vi "Select Popup_General_UI.vi"(8 "error in (no error)":errorcluster, 9 "Self Enqueuer":refnum<class "Message Enqueuer.lvclass">, 11 "ZenGage v3.0 UI in":refnum<class "ZenGage v3.0 UI.lvclass">) -> (0 "error out":errorcluster, 1 "Selection Cancelled?":bool, 2 "JSON Read?":bool, 3 "ZenGage v3.0 UI out":refnum<class "ZenGage v3.0 UI.lvclass">, 5 "Max limits":cluster{"Production max":i32, "Reel max":i32})   [LabVIEW 2015, in "ZenGage v3.0 UI.lvclass"]
uses:
  ZenGage v3.0 UI.lvclass
  <vilib>/ActorFramework/Message Enqueuer/Message Enqueuer.lvclass
  ZenGage v3.0 UI.lvclass/ZenGage v3.0 UI.ctl
  Inspection Statemachine/Inspection Statemachine Messages/Load Selected Part_SM Msg/Load Selected Part_SM Msg.lvclass/Load Selected Part_SM Msg.ctl
  <vilib>/ActorFramework/Message Enqueuer/Message Enqueuer.lvclass/Message Enqueuer.ctl
  <vilib>/ActorFramework/Message Enqueuer/Enqueue.vi
  <vilib>/ActorFramework/Message Priority Queue/Priority Enqueue.vi
  Inspection Statemachine/Inspection Statemachine Messages/Load Selected Part_SM Msg/Load Selected Part_SM Msg.lvclass
panel:
  in  "cancel button":bool
  out "Dialog Box out":string="             SELECT A PART TO INSPECT"
  in  "Combo Box":string(combo)
  in  "String":string
  in  "Numeric Control":dbl
  in  "OK Button":bool
  in  "OK Button":bool
  in  "ORDER NUMBER":dbl
  in  "ORDER NUMBER":dbl
  in  "OPERATOR ID":string
  in  "ORDER NUMBER":dbl
  in  "PART NAME":string(combo)
  # "Select a part to Inspect"
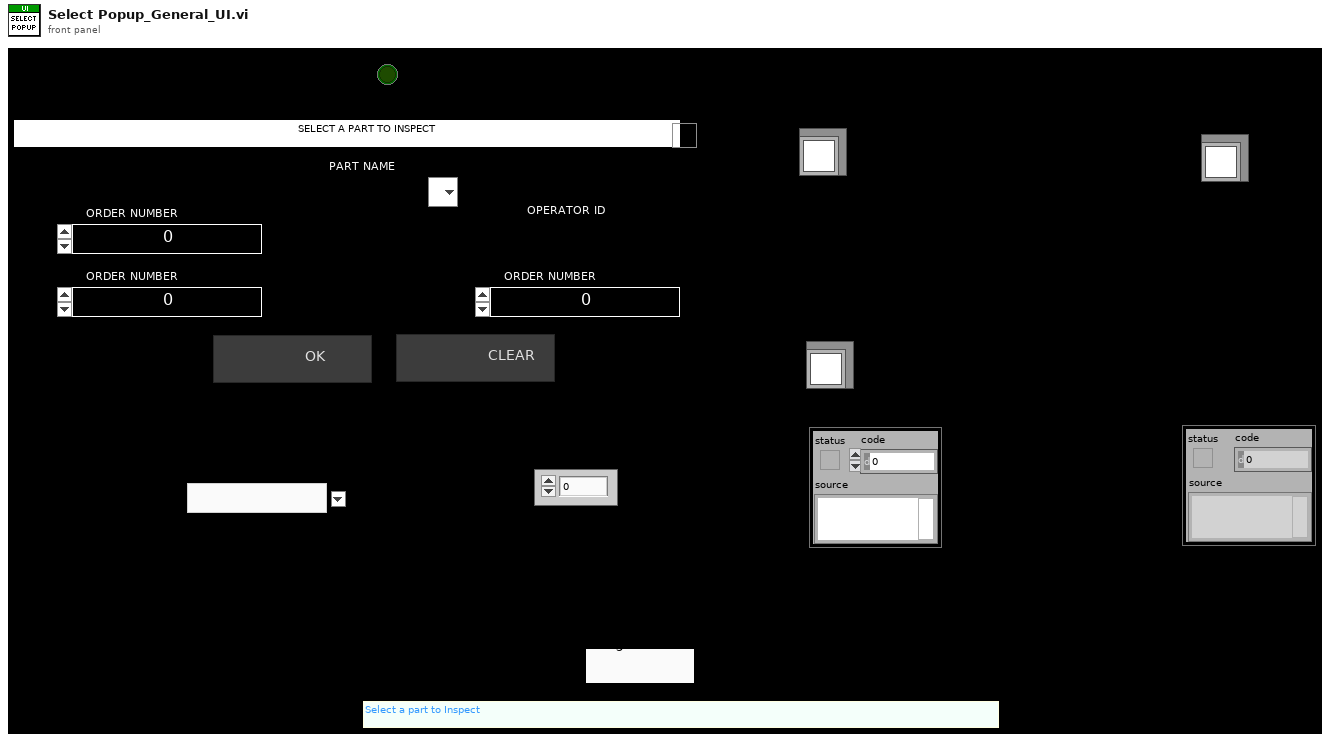
[diagram p1: front panel]
types:
  T1 = enum32{"Invalid", "Standard", "Closed", "Hidden", "Minimized", "Maximized"}
  T2 = cluster{"Part Name":string, "Total Counts":u64, "Connectors in Reel":u64, "Stamping machine ID":u8, "Operator Code":string, "Rack-1 ":bool, "Rack-2 ":bool, "Number of Racks":i32}
  T3 = cluster{"Part Name":string, "Operator Number":string, "Order Number":string}
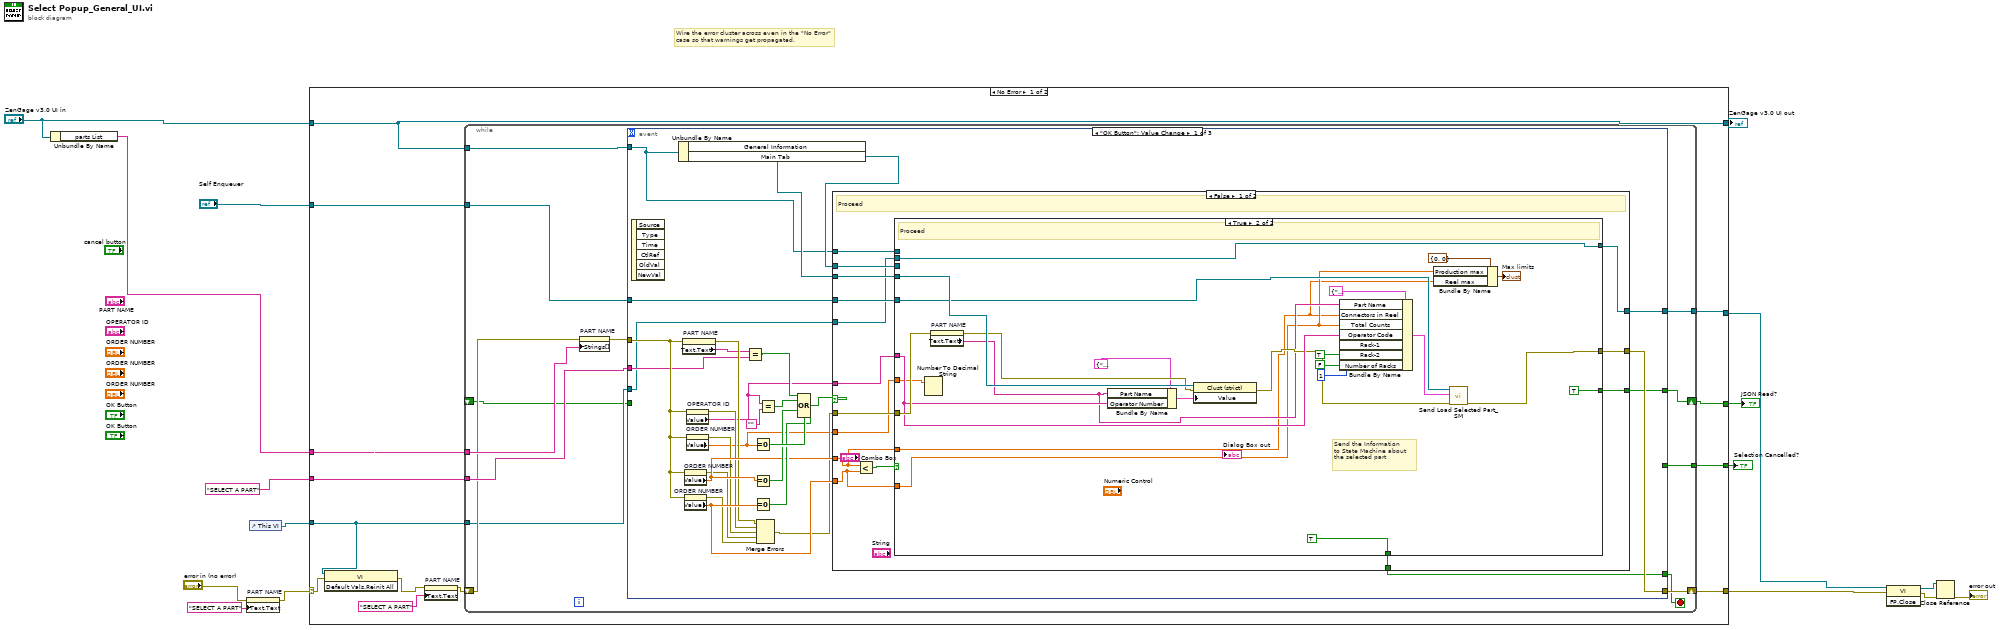
[diagram p0: block diagram]
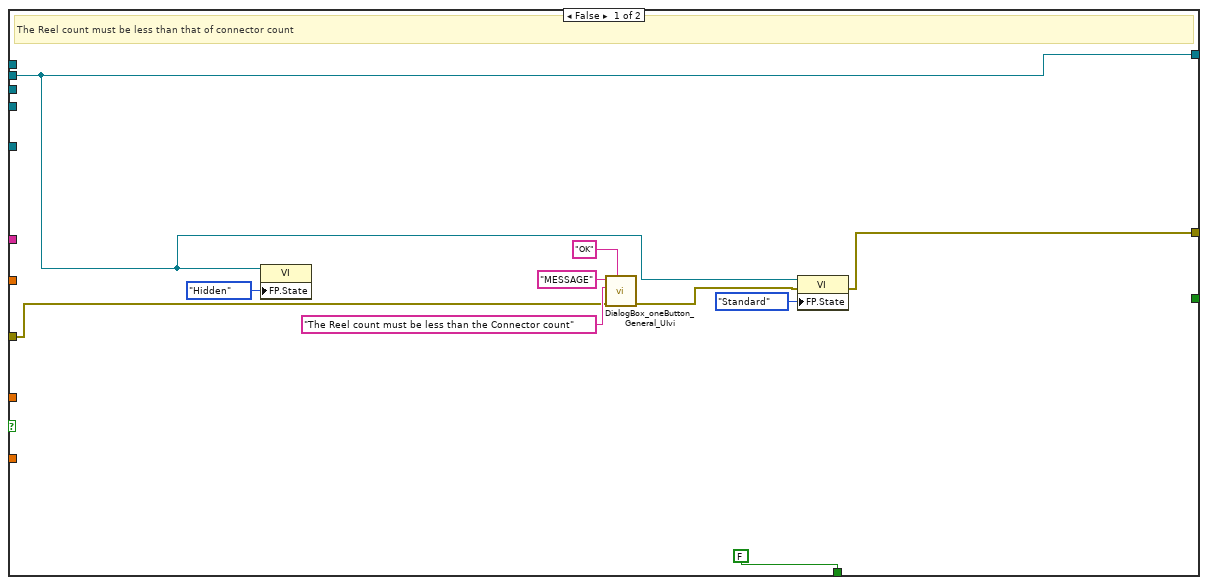
[diagram p2: hidden frame]
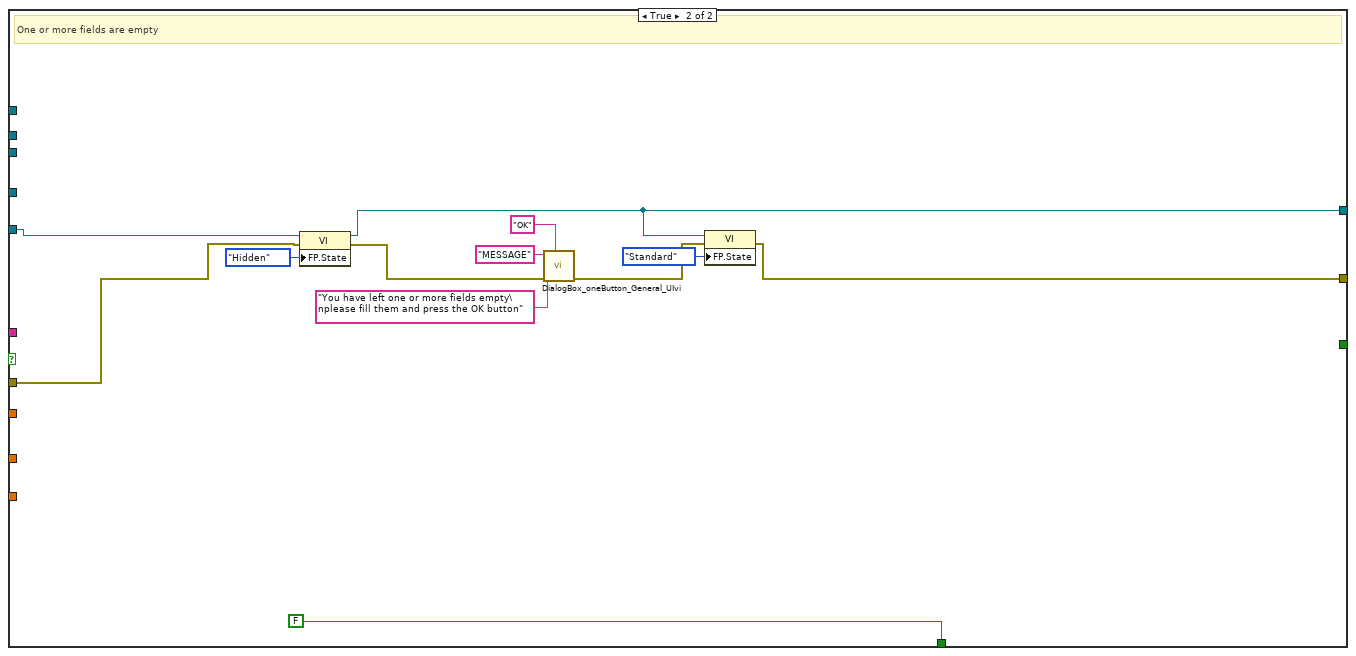
[diagram p3: hidden frame]
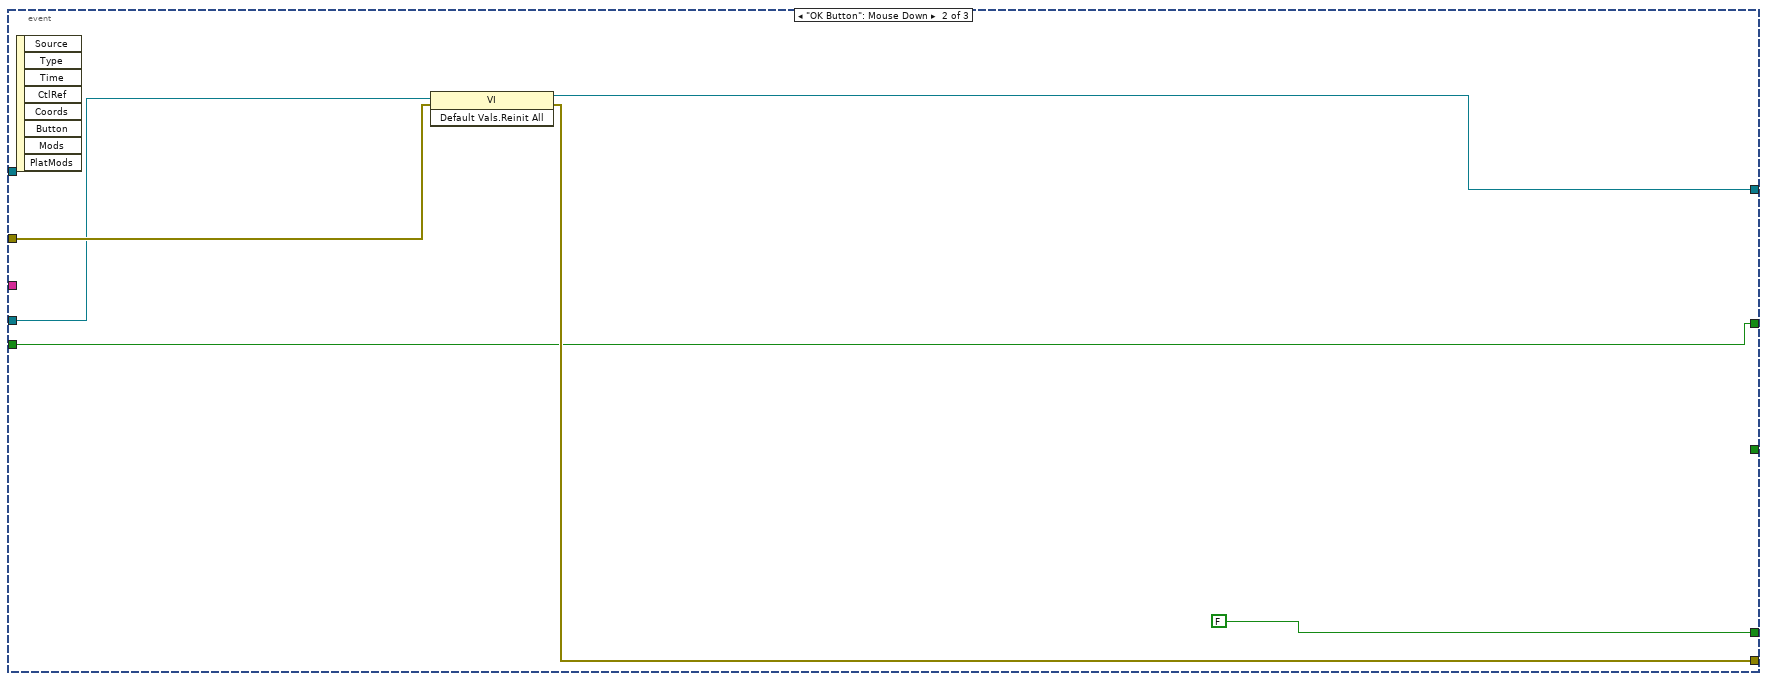
[diagram p4: hidden frame]
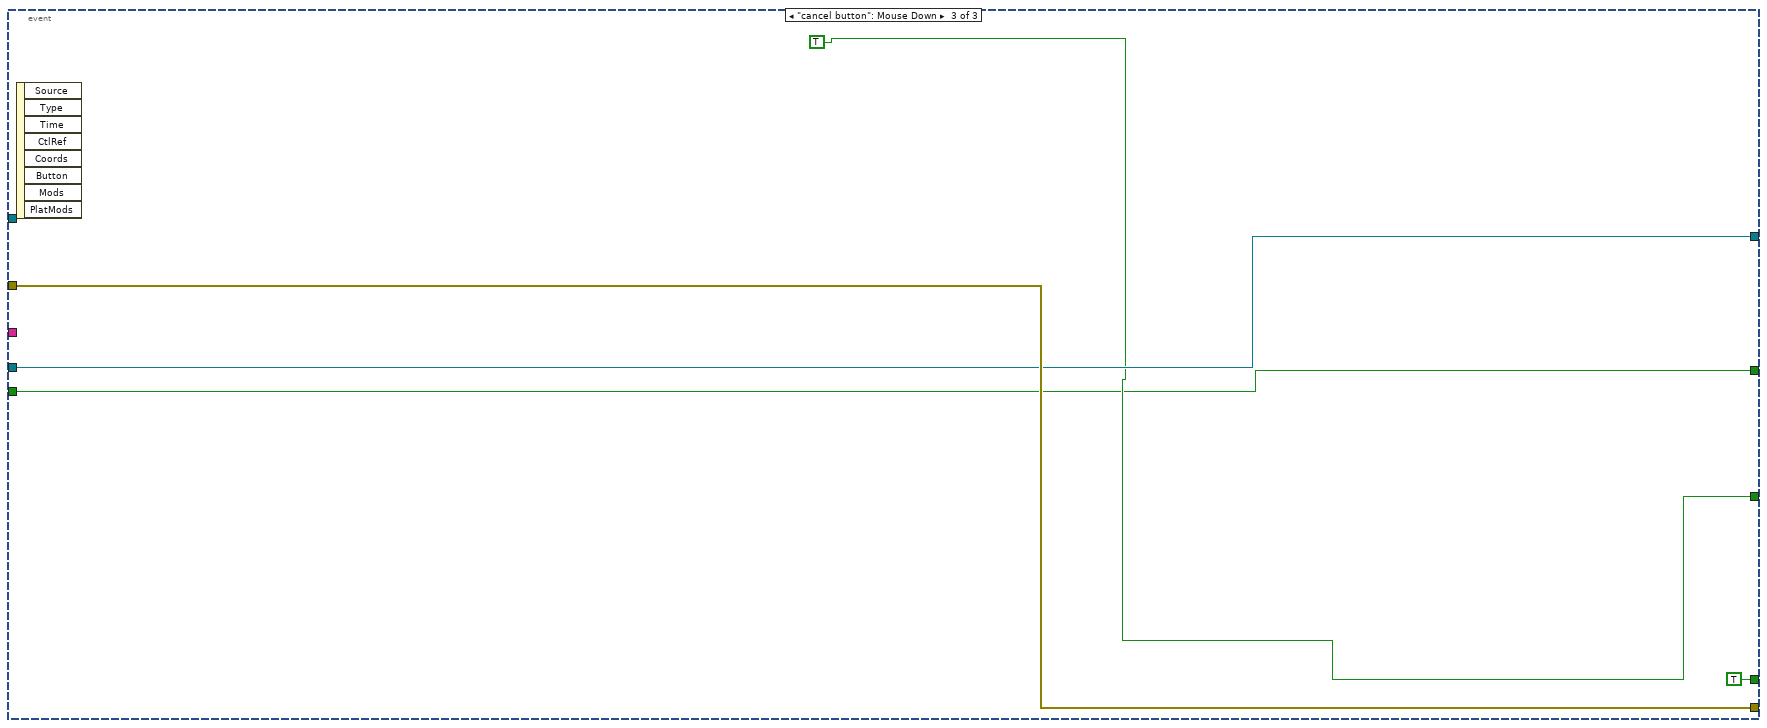
[diagram p5: hidden frame]
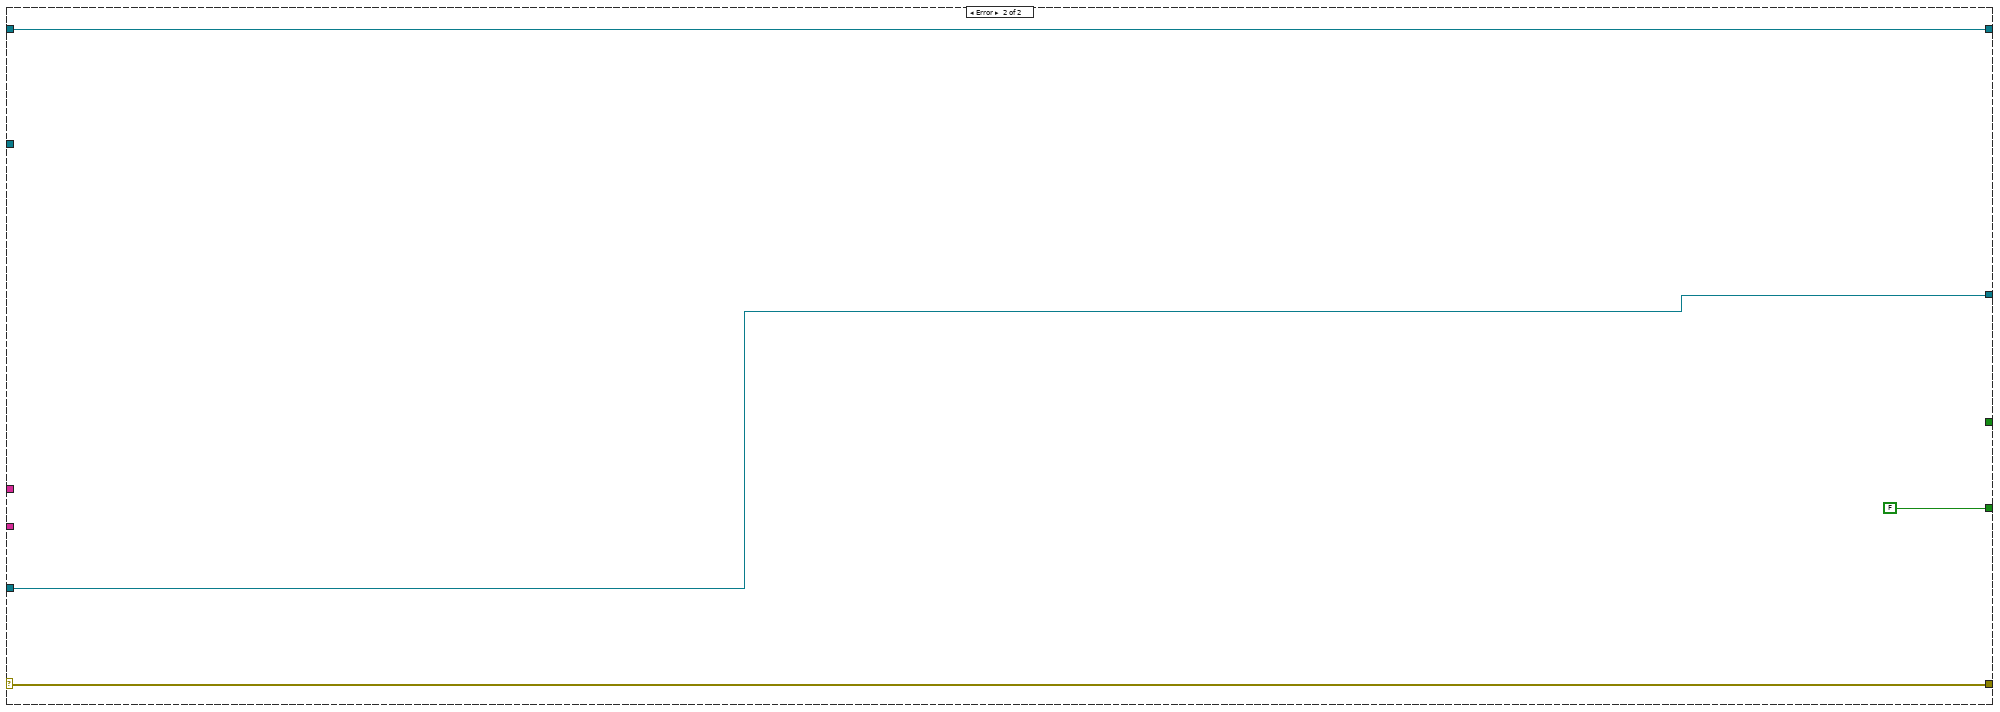
[diagram p6: hidden frame]
diagram:
  # "Wire the error cluster across even in the \"No Error\"\ncase so that warnings get propagated."
  n1 = Unbundle By Name("ZenGage v3.0 UI in") -> ("parts List"=w2:string[])
  n2 = property on="PART NAME" class="CmbBox"(error in="error in (no error)", "Text.Text"="SELECT A PART") -> (error out=w10:errorcluster)  [unwired: 1 in, 1 out]
  n3 = control-ref of="This VI"() -> (w9:refnum<vi>)
  n4 = case shown="No Error" w10 {
    selector: w10 -> [w23 w146]
    tunnel: [w29 w146] -> w5
    tunnel: [w27 w145] -> w16
    tunnel: "ZenGage v3.0 UI in" -> [w27 w145]
    tunnel: w2 -> [w28 _]
    tunnel: "Self Enqueuer" -> [w26 _]
    tunnel: "SELECT A PART" ("new element/subarray") -> [w25 _]
    tunnel: [w24 FALSE] -> w13
    tunnel: [w19 w143] -> w4
    tunnel: w9 -> [w18 w143]
    tunnel: [w17 _] -> w1
    frame No Error {
      n5 = invoke class="VI" method="Default Vals.Reinit All"(reference=w18, error in=w23) -> (error out=w22:errorcluster)  [unwired: 1 in, 2 out]
      n6 = property on="PART NAME" class="CmbBox"(error in=w22, "Text.Text"="SELECT A PART") -> (error out=w21:errorcluster)  [unwired: 1 in, 1 out]
      n7 = while {
        shift-right: [w42] -> w29
        shift-left: w21 -> [w34]
        tunnel: w28 -> [w39]
        tunnel: w27 -> [w40]
        tunnel: w26 -> [w37]
        tunnel: w25 -> [w35]
        tunnel: [w36] -> w24
        tunnel: w18 -> [w33]
        tunnel: [w32] -> w19
        shift-right: [w31] -> w17
        shift-left: _ -> [w30]
        stop <- w41 stop-if-true
        n8 = property on="PART NAME" class="CmbBox"(error in=w34, "Strings[]"=w39) -> (error out=w38:errorcluster)  [unwired: 1 in, 1 out]
        n9 = event shown="[0] \"OK Button\": Value Change" {
          selector: _ -> [_ _ _]
          dyn-events: _ -> [_ _ _]
          timeout: _ -> [_ _ _]
          tunnel: [w65 w135 w142] -> w42
          tunnel: w38 -> [w59 w136 w142]
          tunnel: [w57 FALSE TRUE] -> w41
          tunnel: w40 -> [w51 _ _]
          tunnel: w37 -> [w50 _ _]
          tunnel: w35 -> [w49 _ _]
          tunnel: [_ _ TRUE] -> w36
          tunnel: w33 -> [w45 w134 w141]
          tunnel: [w44 w133 w141] -> w32
          tunnel: [w43 w132 w138] -> w31
          tunnel: w30 -> [_ w132 w138]
          event "OK Button": Value Change {
            n10 = event-data() -> ()  [unwired: 1 in, 6 out]
            n11 = Unbundle By Name(w51) -> ("General Information"=w56:refnum<vi>, "Main Tab"=w52:refnum<vi>)
            n12 = property on="PART NAME" class="CmbBox"(error in=w59) -> (error out=w64:errorcluster, "Text.Text"=w55:string)  [unwired: 1 in, 1 out]
            n13 = property on="ORDER NUMBER" class="DigNum (strict)"(error in=w59) -> (error out=w61:errorcluster, "Value"=w67:dbl)  [unwired: 1 in, 1 out]
            n14 = property on="ORDER NUMBER" class="DigNum (strict)"(error in=w59) -> (error out=w60:errorcluster, "Value"=w66:dbl)  [unwired: 1 in, 1 out]
            n15 = property on="ORDER NUMBER" class="DigNum (strict)"(error in=w59) -> (error out=w62:errorcluster, "Value"=w53:dbl)  [unwired: 1 in, 1 out]
            n16 = property on="OPERATOR ID" class="Str"(error in=w59) -> (error out=w63:errorcluster, "Value"=w48:string)  [unwired: 1 in, 1 out]
            n17 = Equal?(x=w55, y=w49) -> (x = y?=w54:bool)
            n18 = Equal To 0?(x=w53) -> (x = 0?=w71:bool)
            n19 = Equal To 0?(x=w67) -> (x = 0?=w70:bool)
            n20 = Equal To 0?(x=w66) -> (x = 0?=w69:bool)
            n21 = Merge Errors(w64, w63, w62, w61, w60) -> (w58:errorcluster)
            n22 = Equal?(x=w48, y="") -> (x = y?=w46:bool)
            n23 = Compound Arithmetic op=OR(w54, w46, w71, w70, w69) -> (w68:bool)
            n24 = case shown="False" w68 {
              tunnel: w67 -> [w75 _]
              tunnel: w66 -> [w77 _]
              tunnel: w58 -> [w85 w125]
              tunnel: [w84 w121] -> w65
              tunnel: [w80 FALSE] -> w57
              tunnel: w56 -> [w83 _]
              tunnel: w48 -> [w82 _]
              tunnel: w53 -> [w81 _]
              tunnel: w52 -> [w79 _]
              tunnel: w51 -> [w78 _]
              tunnel: w50 -> [w76 _]
              tunnel: w45 -> [w74 w127]
              tunnel: [w73 w120] -> w44
              tunnel: [w72 _] -> w43
              frame False {
                # "Proceed"
                n25 = Less?(x=w75, y=w77) -> (x < y?=w86:bool)
                n26 = case shown="True" w86 {
                  tunnel: w85 -> [w93 w118]
                  tunnel: [w87 w104] -> w84
                  tunnel: w83 -> [_ w119]
                  tunnel: w82 -> [_ w117]
                  tunnel: w81 -> [_ w116]
                  tunnel: [FALSE TRUE] -> w80
                  tunnel: w79 -> [_ _]
                  tunnel: w78 -> [_ _]
                  tunnel: w77 -> [_ w101]
                  tunnel: w75 -> [_ w100]
                  tunnel: w76 -> [_ w112]
                  tunnel: w74 -> [w90 w108]
                  tunnel: [w90 w108] -> w73
                  tunnel: [_ TRUE] -> w72
                  frame False {
                    # "The Reel count must be less than that of connector count"
                    n27 = property class="VI"(reference=w90, "FP.State"=T1."Hidden" ("Front Panel Window:State")) -> ()  [unwired: 1 in, 2 out]
                    n28 = call "DialogBox_oneButton_General_UIvi.vi"("Button Name"="OK" ("Boolean Text.Text"), "error in (no error)"=w93, "Message in"="The Reel count must be less than the Connector count" ("Message Input"), "Dialogbox header"="MESSAGE" ("Dialog Box Input")) -> ("error out"=w88:errorcluster)  [unwired: 6 in, 1 out]
                    n29 = property class="VI"(reference=w90, error in=w88, "FP.State"=T1."Standard" ("Front Panel Window:State")) -> (error out=w87:errorcluster)  [unwired: 1 out]
                  }
                  frame True {
                    # "Send the Information\nto State Machine about\nthe selected part"
                    # "Proceed"
                    n30 = Number To Decimal String(number=w116) -> ()  [unwired: 1 in, 1 out]
                    n31 = property on="PART NAME" class="CmbBox"(error in=w118) -> (error out=w115:errorcluster, "Text.Text"=w111:string)  [unwired: 1 in, 1 out]
                    n32 = Bundle By Name(cluster=T3 {"Part Name"="", "Operator Number"="", "Order Number"=""} ("Value"), "Part Name"=w111, "Operator Number"=w117) -> (w109:T3)
                    n33 = property class="Clust (strict)"(reference=w119, error in=w115, "Value"=w109) -> (error out=w113:errorcluster)  [unwired: 1 out]
                    n34 = Bundle By Name(cluster=T2 {"Part Name"="", "Total Counts"=0, "Connectors in Reel"=0, "Stamping machine ID"=0, "Operator Code"="", "Rack-1 "=FALSE, "Rack-2 "=FALSE, "Number of Racks"=0} ("Part info"), "Part Name"=w111, "Connectors in Reel"=w100, "Total Counts"=w101, "Operator Code"=w117, "Rack-1"=TRUE, "Rack-2"=FALSE, "Number of Racks"=1) -> (w97:T2)
                    n35 = Bundle By Name(cluster=cluster{"Production max":i32, "Reel max":i32} {"Production max"=0, "Reel max"=0} ("Max limits"), "Production max"=w101, "Reel max"=w100) -> (→"Max limits":cluster{"Production max":i32, "Reel max":i32})
                    n36 = call "Send Load Selected Part_SM.vi"("error in (no error)"=w113, "Part info"=w97, "Message Enqueuer"=w112) -> ("error out"=w104:errorcluster)  [unwired: 7 in, 1 out]
                  }
                }
              }
              frame True {
                # "One or more fields are empty"
                n37 = property class="VI"(reference=w127, error in=w125, "FP.State"=T1."Hidden" ("Front Panel Window:State")) -> (reference out=w120:refnum<vi>, error out=w124:errorcluster)
                n38 = call "DialogBox_oneButton_General_UIvi.vi"("Button Name"="OK" ("Boolean Text.Text"), "error in (no error)"=w124, "Message in"="You have left one or more fields empty\nplease fill them and press the OK button" ("Message Input"), "Dialogbox header"="MESSAGE" ("Dialog Box Input")) -> ("error out"=w122:errorcluster)  [unwired: 6 in, 1 out]
                n39 = property class="VI"(reference=w120, error in=w122, "FP.State"=T1."Standard" ("Front Panel Window:State")) -> (error out=w121:errorcluster)  [unwired: 1 out]
              }
            }
          }
          event "OK Button": Mouse Down {
            n40 = event-data() -> ()  [unwired: 1 in, 8 out]
            n41 = invoke class="VI" method="Default Vals.Reinit All"(reference=w134, error in=w136) -> (reference out=w133:refnum<vi>, error out=w135:errorcluster)  [unwired: 1 in, 1 out]
          }
          event "cancel button": Mouse Down {
            n42 = event-data() -> ()  [unwired: 1 in, 8 out]
          }
        }
      }
    }
    frame Error {
    }
  }
  "ZenGage v3.0 UI out" <- w16
  "Selection Cancelled?" <- w13
  "JSON Read?" <- w1
  n43 = invoke class="VI" method="FP.Close"(reference=w4, error in=w5) -> (reference out=w6:refnum<vi>, error out=w8:errorcluster)  [unwired: 1 in, 1 out]
  n44 = Close Reference(reference=w6, error in (no error)=w8) -> (error out=→"error out":errorcluster)
